vi "Get XNET Software To Install.vi"(8 "error in (no error)":errorcluster, 10 "available software components":T1[](array[typedef]) {"component type" items=["standard", "hidden", "system", "unknown", "startup"]}) -> (0 "error out":errorcluster, 1 "found":bool, 2 "xnet software to install":T1[](array[typedef]) {"component type" items=["standard", "hidden", "system", "unknown", "startup", "image"]})   [LabVIEW 2013]
uses:
  <vilib>/nisyscfg/Software 1.2.ctl
  <vilib>/nisyscfg/Component Type.ctl
  <vilib>/nisyscfg/nisyscfg.lvlib
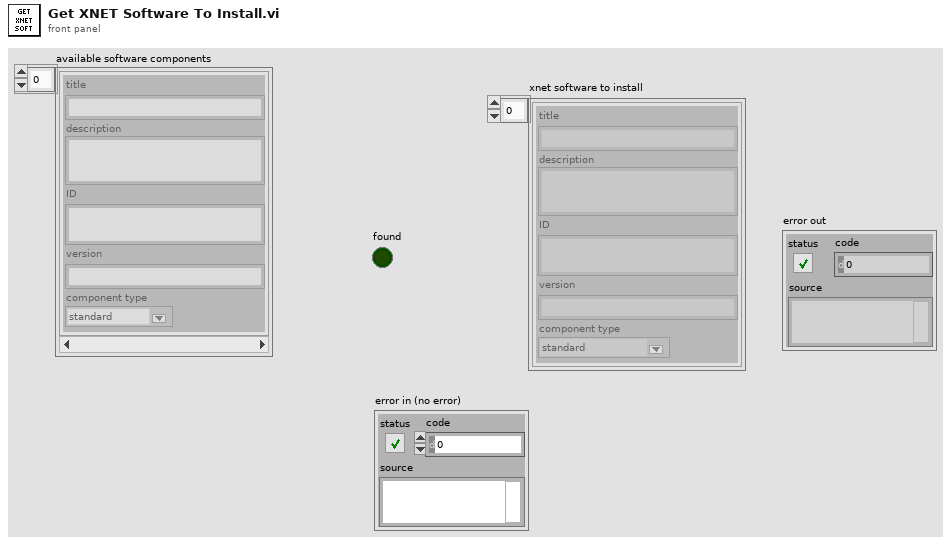
[diagram p1: front panel]
types:
  T1 = typedef "nisyscfg.lvlib/Software 1.2.ctl" = cluster{"title":string, "description":string, "ID":string, "version":string, "component type":T2}
  T2 = typedef "nisyscfg.lvlib/Component Type.ctl" = u32
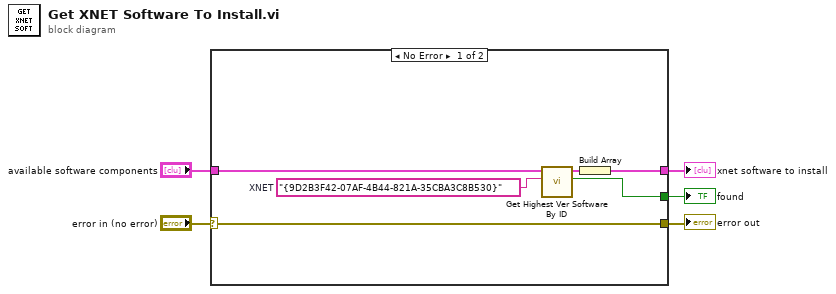
[diagram p0: block diagram]
diagram:
  n1 = case shown="No Error" "error in (no error)" {
    selector: "error in (no error)" -> [w8 w12]
    tunnel: "available software components" -> [w10 _]
    tunnel: [w9 _] -> w3
    tunnel: [w8 w12] -> w2
    tunnel: [w6 _] -> w1
    frame No Error {
      w11 = "{9D2B3F42-07AF-4B44-821A-35CBA3C8B530}"  # XNET
      n2 = call "Get Highest Ver Software By ID.vi"("ID"=w11, "available software components"=w10) -> ("found"=w6:bool, "Software"=w7:T1)  [unwired: 8 in]
      n3 = Build Array(w7) -> (w9:T1[])
    }
    frame Error {
    }
  }
  "xnet software to install" <- w3
  "error out" <- w2
  "found" <- w1
